vi "UHR-Fleezers Control (host) - Lorentz v5.vi"() -> ()   [LabVIEW 2014] (continued)
                                frame #0 {
                                n2596 = property on="Trap Delta (MHz)" class="DigNum (strict)"("Val(Sgnl)"=w3880) -> ()  [unwired: 2 in, 2 out]
                                }
                                frame #1 {
                                n2597 = Wait (ms)(milliseconds to wait=u32 500) -> ()  [unwired: 1 out]
                                }
                                frame #2 {
                                n2598 = local read "Shift confocal"() -> (w3886:bool)
                                n2599 = local read "Mean"() -> (w3887:dbl)
                                n2600 = Greater?(x=w3887, y=11.0) -> (0:w3885:bool)
                                n2601 = And(x=w3885, y=w3886) -> (x .and. y?=w3883:bool)
                                n2602 = Not(x=w3885) -> (.not. x?=w3884:bool)
                                n2603 = And(x=w3884, y=w3886) -> (x .and. y?=w3882:bool)
                                n2604 = case shown="True" w3883 {
                                frame False {
                                }
                                frame True {
                                n2605 = local read "Confocal Y 2 (V)"() -> (w3892:dbl)
                                n2606 = local read "Confocal X 2 (V)"() -> (w3891:dbl)
                                n2607 = property on="AO1" class="Slide (strict)"("Val(Sgnl)"=w3892) -> ()  [unwired: 2 in, 2 out]
                                n2608 = property on="AO2" class="Slide (strict)"("Val(Sgnl)"=w3891) -> ()  [unwired: 2 in, 2 out]
                                }
                                }
                                n2609 = case shown="True" w3882 {
                                frame False {
                                }
                                frame True {
                                n2610 = local read "Confocal Y 1 (V)"() -> (w3890:dbl)
                                n2611 = local read "Confocal X 1 (V)"() -> (w3889:dbl)
                                n2612 = property on="AO2" class="Slide (strict)"("Val(Sgnl)"=w3889) -> ()  [unwired: 2 in, 2 out]
                                n2613 = property on="AO1" class="Slide (strict)"("Val(Sgnl)"=w3890) -> ()  [unwired: 2 in, 2 out]
                                }
                                }
                                }
                                }
                                }
                                }
                                }
                                }
                                }
                                }
                                n2614 = local read "Time (s)"() -> (w3827:dbl)
                                n2615 = Subtract(x=w3828, y=w3827) -> (x-y=w3839:dbl)
                                n2616 = Number To Decimal String(number=w3839, width (-)=i16 0) -> (decimal integer string=w3837:string)
                                n2617 = Concatenate Strings(w3837, " s fluorescence event") -> (w3834:string)
                                n2618 = local read "Messages"() -> (w3835:string)
                                n2619 = local write "Duration (s)"(w3839) -> ()
                                n2620 = call "Update messages.vi"("Message to add"=w3834, "Old message string"=w3835) -> ("New message string"=w3833:string)
                                n2621 = local write "Messages"(w3833) -> ()
                                n2622 = call <vilib>:"Beep.vi"() -> ()  [unwired: 12 in]
                                n2623 = local write "Reset Force"(FALSE ("Force Reset")) -> ()
                                n2624 = local write "Fl. High"(TRUE ("Fl. High")) -> ()
                                n2625 = local write "Waiting"(TRUE ("Waiting")) -> ()
                                }
                                }
                                n2626 = node-c288() -> ()  [unwired: 1 in, 1 out]
                                }
                                n2627 = node-c288(w3806) -> ()  [unwired: 1 out]
                                }
                              }
                            }
                          }
                          n2628 = local read "Trap Delta (MHz)"() -> (w3718:dbl)
                          n2629 = local read "Trap Pos FB SP"() -> (w3716:fxp<+/-,16,1>)
                        }
                      }
                    }
                    frame True {
                      n2630 = flat-sequence {
                        tunnel: w3903 -> [w3913]
                        tunnel: [w3913] -> w3907
                        tunnel: w3906 -> [w3912]
                        tunnel: [w3912] -> w3905
                        tunnel: [w3911] -> w3904
                        tunnel: w3902 -> [w3910]
                        tunnel: [w3909] -> w3901
                        tunnel: w3898 -> [w3908]
                        tunnel: [w3908] -> w3897
                        tunnel: w3907 -> [w3983]
                        tunnel: w3905 -> [w3982]
                        tunnel: w3904 -> [w3981]
                        tunnel: w3901 -> [w3980]
                        tunnel: w3897 -> [w3979]
                        tunnel: [w3980] -> w3900
                        frame #0 {
                          n2631 = call <vilib>:"Beep.vi"() -> ()  [unwired: 3 in, 9 out]
                          n2632 = local write "Waiting"(FALSE ("Waiting")) -> ()
                          n2633 = Increment(x=w3910) -> (x+1=w3909:u8)
                          n2634 = case shown="\"Image\"" w3912 {
                            tunnel: w3909 -> [_ _ w3919]
                            frame "Image" {
                              n2635 = property on="Confocal Image" class="Bool (strict)"("Val(Sgnl)"=TRUE ("Value (Signaling)")) -> ()  [unwired: 2 in, 2 out]
                            }
                            frame "Alarm", Default {
                            }
                            frame "Yank" {
                              n2636 = flat-sequence {
                                tunnel: w3919 -> [w3922]
                                tunnel: [w3921] -> w3918
                                tunnel: ["N Array El"] -> w3917
                                tunnel: w3918 -> [w3936]
                                tunnel: w3917 -> [w3932]
                                frame #0 {
                                n2637 = Multiply(x="Yank Delay (s)", y=1000.0) -> (x*y=w3925:dbl)
                                n2638 = Quotient & Remainder(x=w3922, y="N Array El") -> (x-y*floor(x/y)=w3921:u8)  [unwired: 1 out]
                                n2639 = Wait (ms)(milliseconds to wait=w3925) -> ()  [unwired: 1 out]
                                }
                                frame #1 {
                                n2640 = Random Number (0-1)() -> (number: 0 to 1=w3933:dbl)
                                n2641 = Multiply(x=w3932, y=w3933) -> (x*y=w3931:dbl)
                                n2642 = Round Toward -Infinity(1:w3931) -> (0:w3930:dbl)
                                n2643 = Select(t=w3930, s="Random Choice", f=w3936) -> (s? t:f=w3934:dbl)
                                n2644 = Select(t="Yank to Trap Delta (MHz)", s="Yank to which?", f="Yank to SP") -> (s? t:f=w3927:dbl[])
                                n2645 = Index Array(array=w3927, index=w3934) -> (element=w3937:dbl)
                                n2646 = case shown="False" "Yank to which?" {
                                tunnel: w3937 -> [w3938 w3964]
                                frame False {
                                n2647 = flat-sequence {
                                tunnel: w3938 -> [w3939]
                                frame #0 {
                                n2648 = property on="Trap Pos FB SP" class="DigNum (strict)"("Val(Sgnl)"=w3939) -> ()  [unwired: 2 in, 2 out]
                                }
                                frame #1 {
                                n2649 = Wait (ms)(milliseconds to wait=u32 700) -> ()  [unwired: 1 out]
                                }
                                frame #2 {
                                n2650 = local read "Action (%)"() -> (w3944:dbl)
                                n2651 = Absolute Value(x=w3944) -> (abs(x)=w3943:dbl)
                                n2652 = Greater?(x=w3943, y=70.0) -> (0:w3941:bool)
                                n2653 = property on="Remove Action Offset" class="Bool (strict)"("Val(Sgnl)"=w3941) -> ()  [unwired: 2 in, 2 out]
                                }
                                frame #3 {
                                n2654 = for {
                                N: 4 -> [_]
                                n2655 = flat-sequence {
                                frame #0 {
                                n2656 = Wait (ms)(milliseconds to wait=u32 500) -> ()  [unwired: 1 out]
                                }
                                frame #1 {
                                n2657 = local read "Action (%)"() -> (w3950:dbl)
                                n2658 = Absolute Value(x=w3950) -> (abs(x)=w3949:dbl)
                                n2659 = Greater?(x=w3949, y=70.0) -> (0:w3947:bool)
                                n2660 = property on="Remove Action Offset" class="Bool (strict)"("Val(Sgnl)"=w3947) -> ()  [unwired: 2 in, 2 out]
                                }
                                }
                                }
                                }
                                frame #4 {
                                n2661 = local read "Shift confocal"() -> (w3954:bool)
                                n2662 = local read "Mean"() -> (w3957:dbl)
                                n2663 = Greater?(x=w3957, y=11.0) -> (0:w3953:bool)
                                n2664 = Not(x=w3953) -> (.not. x?=w3952:bool)
                                n2665 = And(x=w3952, y=w3954) -> (x .and. y?=w3951:bool)
                                n2666 = And(x=w3953, y=w3954) -> (x .and. y?=w3955:bool)
                                n2667 = case shown="True" w3955 {
                                frame False {
                                }
                                frame True {
                                n2668 = local read "Confocal X 2 (V)"() -> (w3960:dbl)
                                n2669 = local read "Confocal Y 2 (V)"() -> (w3961:dbl)
                                n2670 = property on="AO2" class="Slide (strict)"("Val(Sgnl)"=w3960) -> ()  [unwired: 2 in, 2 out]
                                n2671 = property on="AO1" class="Slide (strict)"("Val(Sgnl)"=w3961) -> ()  [unwired: 2 in, 2 out]
                                }
                                }
                                n2672 = case shown="True" w3951 {
                                frame False {
                                }
                                frame True {
                                n2673 = local read "Confocal X 1 (V)"() -> (w3958:dbl)
                                n2674 = local read "Confocal Y 1 (V)"() -> (w3959:dbl)
                                n2675 = property on="AO1" class="Slide (strict)"("Val(Sgnl)"=w3959) -> ()  [unwired: 2 in, 2 out]
                                n2676 = property on="AO2" class="Slide (strict)"("Val(Sgnl)"=w3958) -> ()  [unwired: 2 in, 2 out]
                                }
                                }
                                }
                                frame #5 {
                                n2677 = Wait (ms)(milliseconds to wait=u32 1500) -> ()  [unwired: 1 out]
                                }
                                frame #6 {
                                n2678 = property on="Rem fb disp offset" class="Bool (strict)"("Val(Sgnl)"=TRUE ("Value (Signaling)")) -> ()  [unwired: 2 in, 2 out]
                                }
                                }
                                }
                                frame True {
                                n2679 = flat-sequence {
                                tunnel: w3964 -> [w3965]
                                frame #0 {
                                n2680 = property on="Trap Delta (MHz)" class="DigNum (strict)"("Val(Sgnl)"=w3965) -> ()  [unwired: 2 in, 2 out]
                                }
                                frame #1 {
                                n2681 = Wait (ms)(milliseconds to wait=u32 500) -> ()  [unwired: 1 out]
                                }
                                frame #2 {
                                n2682 = local read "Shift confocal"() -> (w3969:bool)
                                n2683 = local read "Mean"() -> (w3967:dbl)
                                n2684 = Greater?(x=w3967, y=11.0) -> (0:w3970:bool)
                                n2685 = Not(x=w3970) -> (.not. x?=w3971:bool)
                                n2686 = And(x=w3971, y=w3969) -> (x .and. y?=w3973:bool)
                                n2687 = And(x=w3970, y=w3969) -> (x .and. y?=w3972:bool)
                                n2688 = case shown="True" w3972 {
                                frame False {
                                }
                                frame True {
                                n2689 = local read "Confocal Y 2 (V)"() -> (w3977:dbl)
                                n2690 = local read "Confocal X 2 (V)"() -> (w3976:dbl)
                                n2691 = property on="AO1" class="Slide (strict)"("Val(Sgnl)"=w3977) -> ()  [unwired: 2 in, 2 out]
                                n2692 = property on="AO2" class="Slide (strict)"("Val(Sgnl)"=w3976) -> ()  [unwired: 2 in, 2 out]
                                }
                                }
                                n2693 = case shown="True" w3973 {
                                frame False {
                                }
                                frame True {
                                n2694 = local read "Confocal X 1 (V)"() -> (w3974:dbl)
                                n2695 = local read "Confocal Y 1 (V)"() -> (w3975:dbl)
                                n2696 = property on="AO2" class="Slide (strict)"("Val(Sgnl)"=w3974) -> ()  [unwired: 2 in, 2 out]
                                n2697 = property on="AO1" class="Slide (strict)"("Val(Sgnl)"=w3975) -> ()  [unwired: 2 in, 2 out]
                                }
                                }
                                }
                                }
                                }
                                }
                                }
                              }
                            }
                          }
                          n2698 = local read "Time (s)"() -> (w3911:dbl)
                          "Fl. High" <- TRUE ("Yanking")
                        }
                        frame #1 {
                          n2699 = local read "Auto F Reset"() -> (w3978:bool)
                          n2700 = case shown="True" w3978 {
                            tunnel: w3983 -> [_ w3987]
                            tunnel: w3982 -> [_ w3986]
                            tunnel: w3981 -> [_ w3985]
                            tunnel: w3979 -> [_ w3984]
                            frame False {
                            }
                            frame True {
                              n2701 = node-c288() -> (w3989:T36)  [unwired: 4 out]
                              n2702 = timed-loop {
                                timing: w3989 -> [_]
                                timing-out: [_] -> w3988
                                tunnel: w3987 -> [w4007]
                                tunnel: w3986 -> [w4006]
                                tunnel: w3985 -> [w4005]
                                tunnel: w3984 -> [w4004]
                                stop <- w3990 stop-if-true
                                n2703 = node-c288() -> ()  [unwired: 2 out]
                                n2704 = local read "Fl. Delta Thresh. (kHz)"() -> (w3998:dbl)
                                n2705 = local read "Fl. Triggered..."() -> (w4003:bool)
                                n2706 = local read "Delta Fl. 1"() -> (w3994:dbl)
                                n2707 = local read "Delta Fl. 2"() -> (w3992:dbl)
                                n2708 = local read "Stop All"() -> (w4001:bool)
                                n2709 = local read "APD to Watch"() -> (w3993:bool)
                                n2710 = Select(t=w3994, s=w3993, f=w3992) -> (s? t:f=w3991:dbl)
                                n2711 = Not(x=w4003) -> (.not. x?=w4002:bool)
                                n2712 = Multiply(x=w3998, y=1000.0) -> (x*y=w3997:dbl)
                                n2713 = Negate(x=w3997) -> (-x=w3996:dbl)
                                n2714 = Less?(x=w3991, y=w3996) -> (x < y?=w4000:bool)
                                n2715 = Compound Arithmetic op=OR(w4000, w4001, w4002, "Reset Force") -> (w3990:bool)
                                n2716 = case shown="True" w3990 {
                                tunnel: w4007 -> [_ w4022]
                                tunnel: w4006 -> [_ w4021]
                                tunnel: w4005 -> [_ w4011]
                                tunnel: w4004 -> [_ w4013]
                                frame False {
                                }
                                frame True {
                                n2717 = local read "Time (s)"() -> (w4012:dbl)
                                n2718 = case shown="\"Yank\"" w4021 {
                                tunnel: w4022 -> [_ w4025]
                                tunnel: w4013 -> [_ w4023]
                                frame "Image", Default {
                                }
                                frame "Yank" {
                                n2719 = flat-sequence {
                                tunnel: [w4031] -> w4026
                                tunnel: w4025 -> [w4031]
                                tunnel: [w4027] -> w4024
                                tunnel: w4023 -> [w4027]
                                tunnel: w4026 -> [w4034]
                                tunnel: w4024 -> [w4032]
                                frame #0 {
                                n2720 = local read "Yank Delay (s)"() -> (w4030:dbl)
                                n2721 = Multiply(x=w4030, y=1000.0) -> (x*y=w4028:dbl)
                                n2722 = Wait (ms)(milliseconds to wait=w4028) -> ()  [unwired: 1 out]
                                }
                                frame #1 {
                                n2723 = local read "Yank to which?"() -> (w4033:bool)
                                n2724 = case shown="False" w4033 {
                                tunnel: w4034 -> [_ w4061]
                                tunnel: w4032 -> [w4035 _]
                                frame False {
                                n2725 = flat-sequence {
                                tunnel: w4035 -> [w4036]
                                frame #0 {
                                n2726 = property on="Trap Pos FB SP" class="DigNum (strict)"("Val(Sgnl)"=w4036) -> ()  [unwired: 2 in, 2 out]
                                }
                                frame #1 {
                                n2727 = Wait (ms)(milliseconds to wait=u32 700) -> ()  [unwired: 1 out]
                                }
                                frame #2 {
                                n2728 = local read "Action (%)"() -> (w4041:dbl)
                                n2729 = Absolute Value(x=w4041) -> (abs(x)=w4040:dbl)
                                n2730 = Greater?(x=w4040, y=70.0) -> (0:w4038:bool)
                                n2731 = property on="Remove Action Offset" class="Bool (strict)"("Val(Sgnl)"=w4038) -> ()  [unwired: 2 in, 2 out]
                                }
                                frame #3 {
                                n2732 = for {
                                N: 4 -> [_]
                                n2733 = flat-sequence {
                                frame #0 {
                                n2734 = Wait (ms)(milliseconds to wait=u32 500) -> ()  [unwired: 1 out]
                                }
                                frame #1 {
                                n2735 = local read "Action (%)"() -> (w4047:dbl)
                                n2736 = Absolute Value(x=w4047) -> (abs(x)=w4046:dbl)
                                n2737 = Greater?(x=w4046, y=70.0) -> (0:w4044:bool)
                                n2738 = property on="Remove Action Offset" class="Bool (strict)"("Val(Sgnl)"=w4044) -> ()  [unwired: 2 in, 2 out]
                                }
                                }
                                }
                                }
                                frame #4 {
                                n2739 = local read "Shift confocal"() -> (w4052:bool)
                                n2740 = local read "Mean"() -> (w4054:dbl)
                                n2741 = Greater?(x=w4054, y=11.0) -> (0:w4051:bool)
                                n2742 = Not(x=w4051) -> (.not. x?=w4050:bool)
                                n2743 = And(x=w4051, y=w4052) -> (x .and. y?=w4049:bool)
                                n2744 = And(x=w4050, y=w4052) -> (x .and. y?=w4048:bool)
                                n2745 = case shown="True" w4049 {
                                frame False {
                                }
                                frame True {
                                n2746 = local read "Confocal Y 2 (V)"() -> (w4058:dbl)
                                n2747 = local read "Confocal X 2 (V)"() -> (w4057:dbl)
                                n2748 = property on="AO2" class="Slide (strict)"("Val(Sgnl)"=w4057) -> ()  [unwired: 2 in, 2 out]
                                n2749 = property on="AO1" class="Slide (strict)"("Val(Sgnl)"=w4058) -> ()  [unwired: 2 in, 2 out]
                                }
                                }
                                n2750 = case shown="True" w4048 {
                                frame False {
                                }
                                frame True {
                                n2751 = local read "Confocal X 1 (V)"() -> (w4055:dbl)
                                n2752 = local read "Confocal Y 1 (V)"() -> (w4056:dbl)
                                n2753 = property on="AO1" class="Slide (strict)"("Val(Sgnl)"=w4056) -> ()  [unwired: 2 in, 2 out]
                                n2754 = property on="AO2" class="Slide (strict)"("Val(Sgnl)"=w4055) -> ()  [unwired: 2 in, 2 out]
                                }
                                }
                                }
                                frame #5 {
                                n2755 = Wait (ms)(milliseconds to wait=u32 1500) -> ()  [unwired: 1 out]
                                }
                                frame #6 {
                                n2756 = property on="Rem fb disp offset" class="Bool (strict)"("Val(Sgnl)"=TRUE ("Value (Signaling)")) -> ()  [unwired: 2 in, 2 out]
                                }
                                }
                                }
                                frame True {
                                n2757 = flat-sequence {
                                tunnel: w4061 -> [w4062]
                                frame #0 {
                                n2758 = property on="Trap Delta (MHz)" class="DigNum (strict)"("Val(Sgnl)"=w4062) -> ()  [unwired: 2 in, 2 out]
                                }
                                frame #1 {
                                n2759 = Wait (ms)(milliseconds to wait=u32 500) -> ()  [unwired: 1 out]
                                }
                                frame #2 {
                                n2760 = local read "Shift confocal"() -> (w4068:bool)
                                n2761 = local read "Mean"() -> (w4070:dbl)
                                n2762 = Greater?(x=w4070, y=11.0) -> (0:w4067:bool)
                                n2763 = Not(x=w4067) -> (.not. x?=w4066:bool)
                                n2764 = And(x=w4067, y=w4068) -> (x .and. y?=w4065:bool)
                                n2765 = And(x=w4066, y=w4068) -> (x .and. y?=w4064:bool)
                                n2766 = case shown="True" w4065 {
                                frame False {
                                }
                                frame True {
                                n2767 = local read "Confocal Y 2 (V)"() -> (w4074:dbl)
                                n2768 = local read "Confocal X 2 (V)"() -> (w4073:dbl)
                                n2769 = property on="AO2" class="Slide (strict)"("Val(Sgnl)"=w4073) -> ()  [unwired: 2 in, 2 out]
                                n2770 = property on="AO1" class="Slide (strict)"("Val(Sgnl)"=w4074) -> ()  [unwired: 2 in, 2 out]
                                }
                                }
                                n2771 = case shown="True" w4064 {
                                frame False {
                                }
                                frame True {
                                n2772 = local read "Confocal Y 1 (V)"() -> (w4072:dbl)
                                n2773 = local read "Confocal X 1 (V)"() -> (w4071:dbl)
                                n2774 = property on="AO2" class="Slide (strict)"("Val(Sgnl)"=w4071) -> ()  [unwired: 2 in, 2 out]
                                n2775 = property on="AO1" class="Slide (strict)"("Val(Sgnl)"=w4072) -> ()  [unwired: 2 in, 2 out]
                                }
                                }
                                }
                                }
                                }
                                }
                                }
                                }
                                }
                                }
                                n2776 = local read "Messages"() -> (w4020:string)
                                n2777 = Subtract(x=w4012, y=w4011) -> (x-y=w4018:dbl)
                                "Duration (s)" <- w4018
                                n2778 = Number To Decimal String(number=w4018, width (-)=i16 0) -> (decimal integer string=w4016:string)
                                n2779 = Concatenate Strings(w4016, " s fluorescence event." ("string")) -> (w4014:string)
                                n2780 = call "Update messages.vi"("Message to add"=w4014, "Old message string"=w4020) -> ("New message string"=w4019:string)
                                n2781 = local write "Reset Force"(FALSE ("Reset Force")) -> ()
                                n2782 = local write "Waiting"(TRUE ("Waiting")) -> ()
                                n2783 = local write "Messages"(w4019) -> ()
                                n2784 = local write "Fl. High"(FALSE ("Fl. High")) -> ()
                                n2785 = call <vilib>:"Beep.vi"() -> ()  [unwired: 3 in, 9 out]
                                }
                                }
                                n2786 = node-c288() -> ()  [unwired: 2 out]
                              }
                              n2787 = node-c288(w3988) -> ()  [unwired: 1 out]
                            }
                          }
                        }
                      }
                      n2788 = local read "Trap Delta (MHz)"() -> (w3903:dbl)
                      n2789 = local read "Trap Pos FB SP"() -> (w3898:fxp<+/-,16,1>)
                    }
                  }
                }
                frame #1 {
                  n2790 = local read "Stop All"() -> (w4084:bool)
                  n2791 = local read "Fl. Triggered..."() -> (w4082:bool)
                  n2792 = Not(x=w4082) -> (.not. x?=w4083:bool)
                  n2793 = Or(x=w4083, y=w4084) -> (x .or. y?=w4081:bool)
                }
              }
              n2794 = case shown="True" w3675 {
                frame False {
                }
                frame True {
                  n2795 = local read "Confocal Y 1 (V)"() -> (w3685:dbl)
                  n2796 = local read "Confocal X 1 (V)"() -> (w3684:dbl)
                  n2797 = property on="AO2" class="Slide (strict)"("Val(Sgnl)"=w3684) -> ()  [unwired: 2 in, 2 out]
                  n2798 = property on="AO1" class="Slide (strict)"("Val(Sgnl)"=w3685) -> ()  [unwired: 2 in, 2 out]
                }
              }
              n2799 = case shown="True" w3675 {
                frame False {
                }
                frame True {
                  w3683 = FALSE ("Fl. High")
                  n2800 = local write "Waiting"(w3683) -> ()
                  n2801 = local write "Fl. High"(w3683) -> ()
                }
              }
              n2802 = node-c288() -> ()  [unwired: 2 out]
            }
            n2803 = node-c288(w3673) -> ()  [unwired: 1 out]
          }
        }
      }
      event "Start assembly line": Value Change {
        n2804 = event-data() -> ()  [unwired: 7 out]
        n2805 = case shown="True" "Start assembly line" {
          tunnel: w4090 -> [_ w4091]
          frame False {
          }
          frame True {
            n2806 = flat-sequence {
              tunnel: w4091 -> [w4096]
              tunnel: [w4095] -> w4093
              tunnel: w4093 -> [w4128]
              tunnel: [w4127] -> w4092
              tunnel: w4092 -> [w4130]
              tunnel: w4091 -> [w4149]
              frame #0 {
                w4094 = TRUE ("Value (Signaling)")
                n2807 = property on="Green Laser ON" class="Bool (strict)"("Val(Sgnl)"=w4094) -> ()  [unwired: 2 in, 2 out]
                "AL Running" <- w4094
              }
              frame #1 {
                n2808 = node-c288() -> (w4098:T36)  [unwired: 4 in]
                n2809 = timed-loop {
                  timing: w4098 -> [_]
                  timing-out: [_] -> w4097
                  tunnel: w4096 -> [w4106]
                  tunnel: [w4101] -> w4095
                  stop <- w4102 stop-if-true
                  n2810 = node-c288() -> ()  [unwired: 1 in, 1 out]
                  n2811 = local read "APD rates cluster"() -> (w4100:T1)
                  n2812 = Multiply(x="Cy3 Fl.  Thresh. (kHz)", y=1000.0) -> (x*y=w4109:dbl)
                  n2813 = Unbundle By Name(w4100) -> ("APD 1 Rate (Hz)"=w4099:dbl)
                  n2814 = Greater?(x=w4099, y=w4109) -> (0:w4105:bool)
                  n2815 = case shown="True" w4105 {
                    tunnel: w4106 -> [_ w4112]
                    tunnel: [TRUE ("Stage Moving") w4111] -> w4104
                    frame False {
                    }
                    frame True {
                      n2816 = flat-sequence {
                        tunnel: w4112 -> [w4117]
                        tunnel: [w4122] -> w4111
                        frame #0 {
                          n2817 = Multiply(x="AL Delay (s)", y=u32 1000) -> (x*y=w4114:u32)
                          n2818 = Wait (ms)(milliseconds to wait=w4114) -> ()  [unwired: 1 out]
                        }
                        frame #1 {
                          n2819 = property on="Green Laser ON" class="Bool (strict)"("Val(Sgnl)"=FALSE ("Value (Signaling)")) -> ()  [unwired: 2 in, 2 out]
                        }
                        frame #2 {
                          # "upper spot"
                          n2820 = local read "Saved Stage Positions"() -> (w4120:dbl[][])
                          n2821 = local write "Stage Moving"(TRUE ("Stage Moving")) -> ()
                          n2822 = call "move to saved stage position.vi"("Stage VISA resource name in"=w4117, "Position"=5, "Saved Stage Positions"=w4120) -> ("error out"=w4118:errorcluster)  [unwired: 1 in, 1 out]
                          n2823 = local write "Stage Control Serial Error"(w4118) -> ()
                        }
                        frame #3 {
                          w4122 = FALSE ("Stage Moving")
                          n2824 = call <vilib>:"Beep.vi"() -> ()  [unwired: 3 in, 9 out]
                          n2825 = local write "Stage Moving"(w4122) -> ()
                        }
                      }
                    }
                  }
                  n2826 = local read "Stop assembly line"() -> (w4101:bool)
                  n2827 = Not(x=w4104) -> (.not. x?=w4103:bool)
                  n2828 = node-c288() -> ()  [unwired: 1 in, 1 out]
                  n2829 = Or(x=w4103, y=w4101) -> (x .or. y?=w4102:bool)
                }
                n2830 = node-c288(w4097) -> ()  [unwired: 1 out]
              }
              frame #2 {
                n2831 = Not(x=w4128) -> (.not. x?=w4127:bool)
                n2832 = case shown="True" w4127 {
                  frame False {
                  }
                  frame True {
                    n2833 = property on="Red Laser ON" class="Bool (strict)"("Val(Sgnl)"=TRUE ("Value (Signaling)")) -> ()  [unwired: 2 in, 2 out]
                  }
                }
              }
              frame #3 {
                n2834 = node-c288() -> (w4132:T36)  [unwired: 4 in]
                n2835 = timed-loop {
                  timing: w4132 -> [_]
                  timing-out: [_] -> w4131
                  tunnel: [w4135] -> _
                  tunnel: w4130 -> [w4135]
                  stop <- "Stop assembly line" stop-if-true
                  n2836 = node-c288() -> ()  [unwired: 1 in, 1 out]
                  n2837 = local read "APD rates cluster"() -> (w4134:T1)
                  n2838 = Multiply(x="Cy5 Fl.  Thresh. (kHz)", y=1000.0) -> (x*y=w4141:dbl)
                  n2839 = Unbundle By Name(w4134) -> ("APD 2 Rate (Hz)"=w4133:dbl)
                  n2840 = Greater?(x=w4133, y=w4141) -> (0:w4138:bool)
                  n2841 = And(x=w4138, y=w4135) -> (x .and. y?=w4136:bool)
                  n2842 = case shown="True" w4136 {
                    frame False {
                    }
                    frame True {
                      n2843 = property on="Green Laser ON" class="Bool (strict)"("Val(Sgnl)"=TRUE ("Value (Signaling)")) -> ()  [unwired: 2 in, 2 out]
                    }
                  }
                  n2844 = node-c288() -> ()  [unwired: 1 in, 1 out]
                }
                n2845 = node-c288(w4131) -> ()  [unwired: 1 out]
              }
              frame #4 {
                w4148 = FALSE ("Value (Signaling)")
                # "lower spot"
                n2846 = local read "Saved Stage Positions"() -> (w4152:dbl[][])
                n2847 = property on="Red Laser ON" class="Bool (strict)"("Val(Sgnl)"=w4148) -> ()  [unwired: 2 in, 2 out]
                n2848 = property on="Green Laser ON" class="Bool (strict)"("Val(Sgnl)"=w4148) -> ()  [unwired: 2 in, 2 out]
                n2849 = local write "Stage Moving"(TRUE ("Stage Moving")) -> ()
                n2850 = local write "Stop assembly line"(FALSE ("Stop assembly line")) -> ()
                n2851 = call "move to saved stage position.vi"("Stage VISA resource name in"=w4149, "Position"=3, "Saved Stage Positions"=w4152) -> ("error out"=w4151:errorcluster)  [unwired: 1 in, 1 out]
                n2852 = local write "Stage Control Serial Error"(w4151) -> ()
              }
              frame #5 {
                w4154 = FALSE ("Stage Moving")
                n2853 = local write "Stage Moving"(w4154) -> ()
                n2854 = local write "AL Running"(w4154) -> ()
                n2855 = call <vilib>:"Beep.vi"() -> ()  [unwired: 3 in, 9 out]
              }
            }
          }
        }
      }
      event "Stop All": Value Change {
        n2856 = event-data() -> ()  [unwired: 7 out]
        n2857 = local read "Stop All"() -> (w4155:bool)
      }
    }
    n2858 = node-c288() -> ()  [unwired: 2 out]
  }
  n2859 = node-c288(w29) -> ()  [unwired: 1 out]
  n2860 = node-c288(w61) -> ()  [unwired: 1 out]
  n2861 = node-c288(w63) -> ()  [unwired: 1 out]
  n2862 = node-c288(w51) -> ()  [unwired: 1 out]
  n2863 = property on="Saved trap pos" class="WFGraph (strict)"("Visible"=FALSE) -> ()  [unwired: 2 in, 2 out]
  n2864 = property on="Trap Delta Graph" class="WFGraph (strict)"("Visible"=TRUE) -> ()  [unwired: 2 in, 2 out]
  n2865 = disable-structure shown="Disabled" {
    disable-tunnel: w54 -> [w4157 _]
    disable-tunnel: w53 -> [w4156 _]
    frame Disabled {
      n2866 = VISA Close(VISA resource name=w4157, error in (no error)=w4156) -> (error out=w4158:errorcluster)
      n2867 = call <vilib>:"Simple Error Handler.vi"("error in (no error)"=w4158) -> ()  [unwired: 1 in, 8 out]
    }
    frame Enabled {
    }
  }
  n2868 = disable-structure shown="Disabled" {
    disable-tunnel: [w4166 _] -> w15
    disable-tunnel: [w4162 _] -> w14
    disable-tunnel: [w4161 _] -> w13
    disable-tunnel: [w4160 _] -> w12
    disable-tunnel: [w4159 _] -> w11
    frame Disabled {
      # "n samples needed for data"
      n2869 = Unbundle By Name("sound format") -> ("sample rate (S/s)"=w4162:dbl)
      n2870 = call <vilib>:"Sound Output Configure.vi"("number of samples/ch"="number of samples/ch", "sample mode"="sample mode", "sound format"="sound format", "device ID"="device ID") -> ("task ID"=w4166:T50)  [unwired: 6 in, 1 out]
      n2871 = local read "DMA Update Period (s)"() -> (w4163:dbl)
      n2872 = Multiply(x=w4163, y=w4162) -> (x*y=w4161:dbl)
      n2873 = for "Sound time base" {
        N: w4161 -> [_]
        tunnel: [w4170] -> w4164 mode=indexing
        i -> [w4170]
      }
      n2874 = Reciprocal(x=w4162) -> (1/x=w4160:dbl)
      n2875 = Multiply(x=w4164, y=w4160) -> (x*y=w4159:dbl[])
    }
    frame Enabled {
    }
  }
  n2876 = timed-loop "Main data acquisition loop (get data, process data for display, and save data to disk)" {
    tunnel: w10 -> [w4244]
    tunnel: w23 -> [w4243]
    tunnel: [w4503] -> w75
    tunnel: [w4498] -> w74
    timing: w68 -> [_]
    timing-out: [_] -> w67
    tunnel: w45 -> [w4410]
    tunnel: [w4300] -> w16
    tunnel: w15 -> [w4299]
    tunnel: w14 -> [w4297]
    tunnel: w13 -> [w4296]
    tunnel: w12 -> [w4295]
    tunnel: w11 -> [w4294]
    stop <- "Stop All" stop-if-true
    w4192 = 2.0
    w4218 = 3276.7
    w4357 = "Initialize"
    # "Cursor control of MCL trap position"
    # "Values for plotting"
    # "Added by Ronen - the limits imposed on amplitudes sent to AOM\nare not explicitly imposed when using intensity feedback. At amplitude of \n~48% FB intensity is ~1.8, if while feedback is on the value passes 1.8, feedback\nis turned off (indication that feedback algorithm overshoots)."
    # "List of channels in order (X or Y only):\nT1 X (mV)\nT2 X (mV)\nT1 X (nm)\nT2 X (nm)\nT1 FX (pN)\nT2 FX (pN)\nPosition Difference (nm)\nAPD1\nAPD2\nAPD3"
    # "T2 sum"
    # "T1 sum"
    n2877 = node-c288() -> ()  [unwired: 2 out]
    n2878 = First Call?() -> (First Call?: T/F=w4370:bool)
    n2879 = Or(x="Reset", y=w4370) -> (x .or. y?=w4371:bool)
    n2880 = Or(x="Start AOD Scan", y="Trap Raster Scan") -> (x .or. y?=w4457:bool)
    n2881 = case "Reset data stream (manual reset or at begining of some rastering and imaging)" shown="True" w4371 {
      tunnel: w4244 -> [w5254 w5262]
      tunnel: w4243 -> [w5253 w5261]
      tunnel: [w5254 w5256] -> w4274
      tunnel: [w5253 w5255] -> w4275
      frame False {
      }
      frame True {
        w5259 = TRUE ("AI to FIFO")
        n2882 = call "reset FPGA DMA.vi"("error in"=w5261, "FPGA VI Reference In"=w5262) -> ("error out"=w5257:errorcluster, "FPGA VI Reference Out"=w5258:T35)
        n2883 = local write "Overflow (data lost)"(FALSE ("Overflow (data lost)")) -> ()
        n2884 = xnode "Read/Write Control"("FPGA VI Reference In"=w5258, "error in"=w5257, "AI to FIFO"=w5259, "APD to FIFO"=w5259) -> ("FPGA VI Reference Out"=w5256:T35, "error out"=w5255:errorcluster)
      }
    }
    n2885 = case "Start active calibration (oscillate traps precisely)" shown="True" "Active Cal" {
      tunnel: w4275 -> [w4604 w4612]
      tunnel: w4274 -> [w4603 w4613]
      tunnel: [w4604 w4609] -> w4273
      tunnel: [w4603 w4610] -> w4272
      frame False {
      }
      frame True {
        w4605 = TRUE ("APD to FIFO")
        n2886 = call "reset FPGA DMA.vi"("error in"=w4612, "FPGA VI Reference In"=w4613) -> ("error out"=w4606:errorcluster, "FPGA VI Reference Out"=w4607:T35)
        n2887 = local write "Active Cal"(FALSE ("Active Cal")) -> ()
        n2888 = local write "Save Calibration"(TRUE ("Save Calibration")) -> ()
        n2889 = xnode "Read/Write Control"("FPGA VI Reference In"=w4607, "error in"=w4606, "AI to FIFO"=w4605, "APD to FIFO"=w4605) -> ("FPGA VI Reference Out"=w4610:T35, "error out"=w4609:errorcluster)
      }
    }
    n2890 = case shown="True" "Read Lateness and Rel Phase" {
      tunnel: w4244 -> [w4828 w4859]
      tunnel: w4243 -> [w4829 w4858]
      tunnel: [w4828 w4830] -> w4214
      tunnel: [w4829 w4831] -> w4446
      frame False {
      }
      frame True {
        n2891 = xnode "Read/Write Control"("FPGA VI Reference In"=w4859, "error in"=w4858) -> ("FPGA VI Reference Out"=w4830:T35, "error out"=w4831:errorcluster, "GI Relative phase"=→"GI relative phase":i16, "Relative phase"=→"Relative phase (AI1)":i16, "AI Late Counter"=→"Late Counter (AI1)":u8, "GI Late Counter"=→"GI Late Counter":u8, "MCL Late Counter"=→"MCL Late Counter":u8, "MCL Relative Phase"=→"Relative Phase (MCL)":i16, "APD Acq Relative Phase"=→"APD Acq Relative Phase":i16, "APD 1 Gate Relative Phase"=→"APD 1 Gate Relative Phase":i16, "APD 2 Gate Relative Phase"=→"APD 2 Gate Relative Phase":i16, "APD Acq Late Counter"=→"APD Acq Late Counter":u8, "APD 1 Gate Late Counter"=→"APD 1 Gate Late Counter":u8, "APD 2 Gate Late Counter"=→"APD 2 Gate Late Counter":u8, "Green FB Relative Phase"=→"Relative phase (Green FB)":i16, "GI Relative phase 2"=→"GI relative phase 2":i16, "GI Late Counter 2"=→"GI Late Counter 2":u8, "Trap Pos FIFO Timeout"=→"Trap Pos FIFO Timeout":u16, "Trap AI FIFO Timeout"=→"Trap AI FIFO Timeout":u16, "RI Late Counter"=→"RI Late Counter":u8, "RI Relative phase"=→"RI relative phase":i16, "Green Late Counter"=→"Green AI Late Counter":u8, "BI Late Counter (AO)"=→"Late Counter (BI AO)":u8, "Blue Late Counter (D)"=→"Late Counter (BI DO)":u8, "BI Relative phase (AO)"=→"Relative phase (BI AO)":i16, "BI Relative phase (D)"=→"Relative phase (BI DO)":i16, "APD 3 Gate Late Counter"=→"APD 3 Gate Late Counter":u8, "APD 3 Gate Relative Phase"=→"APD 3 Gate Relative Phase":i16)
      }
    }
    n2892 = Compound Arithmetic op=OR("Start MCL Scan", "Confocal Image", "Confocal Linescan") -> (w4242:bool)
    n2893 = And(x="Save Data (MCL)", y=w4242) -> (x .and. y?=w4476:bool)
    n2894 = case "Start AOM raster scan" shown="True" w4457 {
      tunnel: w4272 -> [w5113 w5123]
      tunnel: w4273 -> [w5112 w5122]
      tunnel: [w5113 w5116] -> w4479
      tunnel: [w5112 w5115] -> w4478
      frame False {
      }
      frame True {
        n2895 = case shown="True" "Restart DMA? (AOD)" {
          tunnel: [w5152 w5154] -> w5117
          tunnel: [w5151 w5153] -> w5118
          tunnel: w5123 -> [w5152 w5156]
          tunnel: w5122 -> [w5151 w5155]
          frame False {
          }
          frame True {
            n2896 = local write "Overflow (data lost)"(FALSE ("Overflow (data lost)")) -> ()
            n2897 = call "reset FPGA DMA.vi"("error in"=w5155, "FPGA VI Reference In"=w5156) -> ("error out"=w5153:errorcluster, "FPGA VI Reference Out"=w5154:T35)
          }
        }
        n2898 = local write "Trap Raster Scan"(FALSE ("Trap Raster Scan")) -> ()
        n2899 = case shown="True" "Move MCL Also?" {
          tunnel: w5118 -> [w5126 w5146]
          tunnel: w5117 -> [w5127 w5147]
          tunnel: [w5125 w5150] -> w5116
          tunnel: [w5124 w5149] -> w5115
          frame False {
            w5128 = TRUE ("AI to FIFO")
            n2900 = xnode "Read/Write Control"("FPGA VI Reference In"=w5127, "error in"=w5126, "AI to FIFO"=w5128, "APD to FIFO"=w5128, "Start scan"=w5128) -> ("FPGA VI Reference Out"=w5125:T35, "error out"=w5124:errorcluster)
          }
          frame True {
            w5144 = FALSE ("1D or 2D Scan?")
            w5148 = TRUE ("AI to FIFO")
            n2901 = local read "Scan Range (nm)"() -> (w5141:dbl)
            n2902 = local read "Scan steps (AOD)"() -> (w5135:u64)
            n2903 = local read "Total Counts (ticks)"() -> (w5136:u16)
            n2904 = local read "Cycles/step (AOD)"() -> (w5134:u64)
            n2905 = local read "Number of F/B Scans (AOD)"() -> (w5143:u16)
            n2906 = Bundle("Scan Range (nm)"=w5141, "MCL Step Position Ratio"="MCL Step Position Ratio", "MCL/AOM Scale Tweak"="MCL/AOM Scale Tweak", "MCL X Cal (nm/V)"="MCL X Cal (nm/V)", "MCL Step Increment (V_int)"="MCL Step Increment (V_int)", "Total Counts (ticks)"=w5136, "Scan steps (AOD)"=w5135, "Cycles/step (AOD)"=w5134) -> (w5133:T57)  [unwired: 1 in]
            n2907 = call "Calculate MCL scan parameters.vi"("Input parameters"=w5133) -> ("Scan steps(MCL)"=w5132:dbl, "Scan Freq. Increment (MCL)"=w5131:dbl, "MCL Count"=w5130:dbl)
            "MCL Count" <- w5130
            n2908 = xnode "Read/Write Control"("FPGA VI Reference In"=w5147, "error in"=w5146, "Scan steps (MCL)"=w5132, "Number of scans (MCL)"=w5143, "Cycles per step (MCL)"=u64 1, "Scan freq.  increment (MCL)"=w5131, "1D or 2D Scan?"=w5144, "MCL Scan Axis"=w5144, "Cont. Scan (MCL)"=w5144, "MCL count"=w5130) -> ("FPGA VI Reference Out"=w5129:T35, "error out"=w5145:errorcluster)
            n2909 = local write "MCL Scanning"(w5148) -> ()
            n2910 = local write "wait to reset values"(w5148) -> ()
            n2911 = xnode "Read/Write Control"("FPGA VI Reference In"=w5129, "error in"=w5145, "AI to FIFO"=w5148, "APD to FIFO"=w5148, "Start scan"=w5148, "Start scan (MCL)"=w5148) -> ("FPGA VI Reference Out"=w5150:T35, "error out"=w5149:errorcluster)
          }
        }
        "Raster Scanning..." <- TRUE ("Scanning...")
      }
    }
    n2912 = case "Start MCL raster scan" shown="True" w4242 {
      tunnel: w4479 -> [w5041 w5056]
      tunnel: w4478 -> [w5040 w5055]
      tunnel: [w5041 w5051] -> w4409
      tunnel: [w5040 w5050] -> w4408
      tunnel: [FALSE w5049] -> w4462
      tunnel: "Start MCL Scan" -> [_ w5044]
      tunnel: "Confocal Image" -> [_ w5043]
      tunnel: "Confocal Linescan" -> [_ _]
      frame False {
      }
      frame True {
        w5049 = TRUE
        n2913 = case shown="True" "Restart DMA? (MCL)" {
          tunnel: [w5085 w5087] -> w5054
          tunnel: [w5084 w5086] -> w5053
          tunnel: w5056 -> [w5085 w5090]
          tunnel: w5055 -> [w5084 w5089]
          frame False {
          }
          frame True {
            n2914 = call "reset FPGA DMA.vi"("error in"=w5089, "FPGA VI Reference In"=w5090) -> ("error out"=w5086:errorcluster, "FPGA VI Reference Out"=w5087:T35)
            n2915 = local write "Overflow (data lost)"(FALSE ("Overflow (data lost)")) -> ()
          }
        }
        n2916 = case shown="False" w5044 {
          tunnel: w5043 -> [w5059 _]
          frame False {
            n2917 = property on="Confocal Image" class="Bool (strict)"("Value"=FALSE ("Start Confocal Map")) -> ()  [unwired: 2 in, 2 out]
            n2918 = property on="2D or 1D Scan" class="Bool (strict)"("Val(Sgnl)"=w5059) -> ()  [unwired: 2 in, 2 out]
          }
          frame True {
          }
        }
        n2919 = local write "Tab Control 6"(T3."Imaging" ("Tab Control 6")) -> ()
        n2920 = local write "MCL Scanning"(w5049) -> ()
        n2921 = local read "AO2"() -> (w5045:dbl)
        n2922 = local read "AO1"() -> (w5046:dbl)
        n2923 = case shown="True" "Center Scan" {
          tunnel: w5054 -> [w5066 w5083]
          tunnel: w5053 -> [w5065 w5082]
          tunnel: [w5064 w5081] -> w5051
          tunnel: [w5063 w5080] -> w5050
          tunnel: [w5061 w5068] -> w5048
          tunnel: [w5060 w5067] -> w5047
          tunnel: w5046 -> [w5061 w5073]
          tunnel: w5045 -> [w5060 w5072]
          frame False {
            w5062 = TRUE ("AI to FIFO")
            n2924 = xnode "Read/Write Control"("FPGA VI Reference In"=w5066, "error in"=w5065, "AI to FIFO"=w5062, "APD to FIFO"=w5062, "Start scan (MCL)"=w5062) -> ("FPGA VI Reference Out"=w5064:T35, "error out"=w5063:errorcluster)
          }
          frame True {
            w5079 = TRUE ("AI to FIFO")
            n2925 = local read "Actual MCL Inc (V)"() -> (w5076:dbl)
            n2926 = local read "Scan steps (MCL)"() -> (w5075:u64)
            n2927 = local read "Scan lines (y)"() -> (w5074:u64)
            n2928 = local read "2D or 1D Scan"() -> (w5069:bool)
            n2929 = local read "Fast Scan Dir"() -> (w5070:bool)
            n2930 = Bundle("Actual MCL Inc (V)"=w5076, "Scan steps (MCL)"=w5075, "Scan lines (y)"=w5074, "AO1"=w5073, "AO2"=w5072) -> (w5071:T58)  [unwired: 1 in]
            n2931 = call "Center Scan calculation.vi"("2D or 1D Scan"=w5069, "Fast Scan Dir"=w5070, "Input parameters"=w5071) -> ("AO2"=w5067:dbl, "AO1"=w5068:dbl)
            n2932 = call "Volt to I16.vi"("Voltage In"=w5068) -> ("I16 Voltage Out"=w5078:i16)
            n2933 = call "Volt to I16.vi"("Voltage In"=w5067) -> ("I16 Voltage Out"=w5077:i16)
            n2934 = xnode "Read/Write Control"("FPGA VI Reference In"=w5083, "error in"=w5082, "AI to FIFO"=w5079, "APD to FIFO"=w5079, "Start scan (MCL)"=w5079, "AO1"=w5078, "AO2"=w5077) -> ("FPGA VI Reference Out"=w5081:T35, "error out"=w5080:errorcluster)
          }
        }
        "Initial Y" <- w5048
        "Initial X" <- w5047
        "wait to reset values" <- w5049
      }
    }
    n2935 = xnode "Read/Write Control"("FPGA VI Reference In"=w4214) -> ("FPGA VI Reference Out"=w4173:T35, "BD1 Frequency Out 1"=w4216:u64)  [unwired: 1 in, 1 out]
    n2936 = And(x="Save scans", y=w4457) -> (x .and. y?=w4477:bool)
    n2937 = call "IR AOM word to freq.vi"("Frequency Word In (U64)"=w4216) -> ("Frequency Out (MHz)"=w4215:dbl)
    n2938 = local read "BD 1 Frequency 2 (MHz)"() -> (w4257:dbl)
    n2939 = Subtract(x=w4257, y=w4215) -> (x-y=w4250:dbl)
    "Current deltaF (MHz)" <- w4250
    n2940 = control-ref of="Piezo trap cursor control"() -> (w4174:refnum<vi>)
    n2941 = Unbundle By Name("Cursor control") -> ("X"=w4176:bool, "Y"=w4175:bool)
    n2942 = local read "APD Elements/DMA read"() -> (w4314:u32)
    n2943 = local read "Trap AI Elements/DMA read"() -> (w4444:u32)
    n2944 = case shown="False" w4176 {
      tunnel: w4174 -> [w4530 w4540]
      tunnel: w4173 -> [_ w4532]
      frame False {
        n2945 = local read "T3 X (V)"() -> (w4531:dbl)
        n2946 = property class="XYGraph (strict)"(reference=w4530, "Cursor.Cursor X"=w4531) -> ()  [unwired: 1 in, 2 out]
      }
      frame True {
        n2947 = property class="XYGraph (strict)"(reference=w4540) -> ("Cursor.Cursor X"=w4537:dbl)  [unwired: 1 in, 2 out]
        n2948 = In Range and Coerce(upper limit=10.0, x=w4537, lower limit=0.0) -> (coerced(x)=w4535:dbl)  [unwired: 1 out]
        n2949 = Multiply(x=3276.7, y=w4535) -> (x*y=w4534:dbl)
        n2950 = To Unsigned Word Integer(number=w4534) -> (unsigned 16bit integer=w4533:u16)
        n2951 = xnode "Read/Write Control"("FPGA VI Reference In"=w4532, "Piezo Trap X (AO5)"=w4533) -> ()  [unwired: 1 in, 2 out]
      }
    }
    n2952 = case shown="False" w4175 {
      tunnel: w4174 -> [w4517 w4529]
      tunnel: w4173 -> [_ w4520]
      frame False {
        n2953 = local read "T3 Y (V)"() -> (w4519:dbl)
        n2954 = Negate(x=w4519) -> (-x=w4518:dbl)
        n2955 = property class="XYGraph (strict)"(reference=w4517, "Cursor.Cursor Y"=w4518) -> ()  [unwired: 1 in, 2 out]
      }
      frame True {
        n2956 = property class="XYGraph (strict)"(reference=w4529) -> ("Cursor.Cursor Y"=w4526:dbl)  [unwired: 1 in, 2 out]
        n2957 = In Range and Coerce(upper limit=0.0, x=w4526, lower limit=-10.0) -> (coerced(x)=w4525:dbl)  [unwired: 1 out]
        n2958 = Negate(x=w4525) -> (-x=w4523:dbl)
        n2959 = Multiply(x=3276.7, y=w4523) -> (x*y=w4522:dbl)
        n2960 = To Unsigned Word Integer(number=w4522) -> (unsigned 16bit integer=w4521:u16)
        n2961 = xnode "Read/Write Control"("FPGA VI Reference In"=w4520, "Piezo Trap Y (AO4)"=w4521) -> ()  [unwired: 1 in, 2 out]
      }
    }
    n2962 = local read "Trap Pos Elements/DMA read"() -> (w4405:u32)
    n2963 = local read "DMA Update Period (s)"() -> (w4235:dbl)
    n2964 = xnode "Invoke Method"("FPGA VI Reference In"=w4409, "error in"=w4408, "Number of Elements"=w4405, "Timeout (ms)"=-1) -> ("Data"=w4377:u16[], "Elements Remaining"=→"Trap Pos FIFO El Remaining":u32)  [unwired: 2 out]
    n2965 = xnode "Get Trap Data"("FPGA VI Reference In"=w4409, "error in"=w4408, "Number of Elements"=w4444, "Timeout (ms)"=-1 ("Timeout")) -> ("FPGA VI Reference Out"=w4256:T35, "error out"=w4347:errorcluster, "Data"=w4239:i16[], "Elements Remaining"=w4511:u32)
    "FIFO El. Rem." <- w4511
    n2966 = local read "Trap AI FIFO Depth"() -> (w4513:u32)
